vi "GetUnitsFromString.vi"(8 "error in (no error)":errorcluster, 11 "input string":string) -> (0 "error out":errorcluster, 3 "result string":string)   [LabVIEW 2017]
doc: "Use this template to build a VI to use as a subVI."
uses:
  <vilib>/regexp/Match Regular Expression.xnode
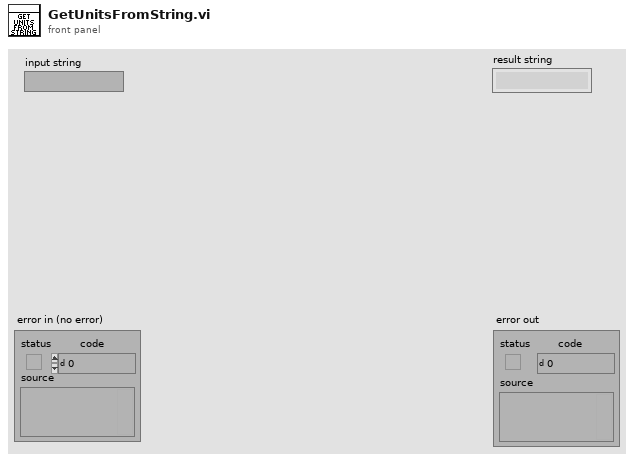
[diagram p1: front panel]
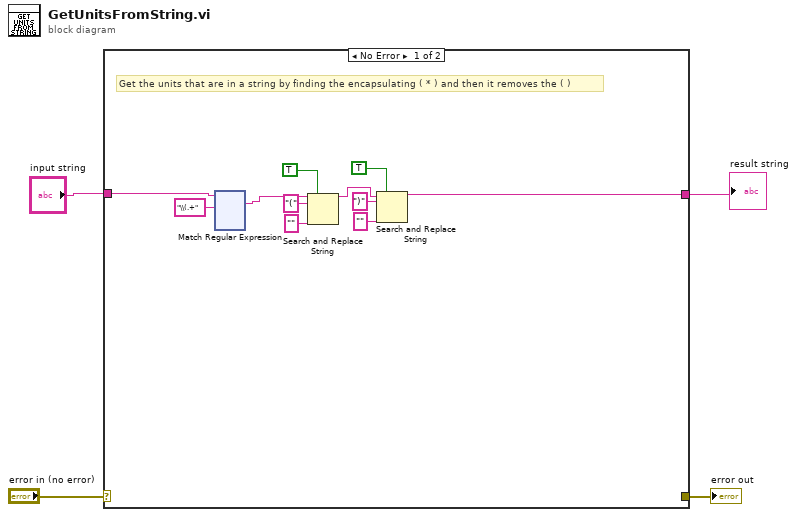
[diagram p0: block diagram]
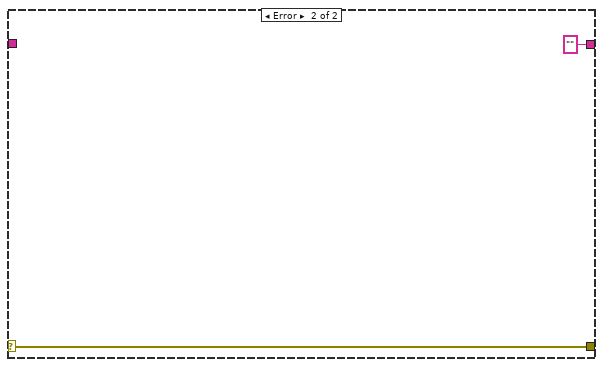
[diagram p2: hidden frame]
diagram:
  n1 = case shown="No Error" "error in (no error)" {
    selector: "error in (no error)" -> [_ w131]
    tunnel: [_ w131] -> w3
    tunnel: [w6 "" ("result string")] -> w2
    tunnel: "input string" -> [w5 _]
    frame No Error {
      # "Get the units that are in a string by finding the encapsulating ( * ) and then it removes the ( )"
      n2 = xnode "Match Regular Expression"("input string"=w5, "regular expression"="\\(.+") -> ("whole match"=w7:string)  [unwired: 4 in, 4 out]
      n3 = Search and Replace String(replace all?=TRUE ("replace all? (F)"), input string=w7, search string="(", replace string="" ("replace string (\"\")")) -> (result string=w14:string)  [unwired: 4 in, 3 out]
      n4 = Search and Replace String(replace all?=TRUE ("replace all? (F)"), input string=w14, search string=")", replace string="" ("replace string (\"\")")) -> (result string=w6:string)  [unwired: 4 in, 3 out]
    }
    frame Error {
    }
  }
  "error out" <- w3
  "result string" <- w2
